vi "Append Image.vi"(1 "Cell Address":string, 4 "Image Path":path, 6 "error in (no error)":errorcluster, 7 "Column Index":i32, 8 "Caption":string, 9 "Row Index":i32, 10 "Report Ref In":T2) -> (0 "error out":errorcluster, 2 "Image Index":i32, 3 "Report Ref Out":T2)   [LabVIEW 2026, in "XCel Report Engine.lvlib"]
uses:
  XCel Report Engine.lvlib
  Controls/Report Ref.ctl
  C:/Users/m.santucci/Documents/ChatGPT/LV_REPORT_ENGINE/.net/src/XCelReportEngine/bin/Release/net48/XCelReportEngine.dll
  .net/src/XCelReportEngine/bin/Release/net48/XCelReportEngine.dll
  Controls/Image Alignment.ctl
panel:
  in  "Image Alignment":T1
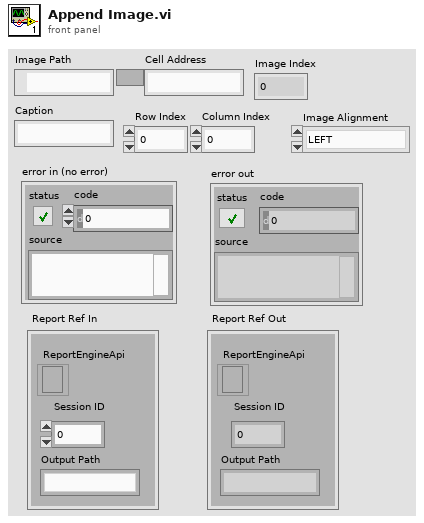
[diagram p1: front panel]
types:
  T1 = typedef "XCel Report Engine.lvlib/Image Alignment.ctl" = enum32{"LEFT", "RIGHT", "TOP", "TEXTTOP", "MIDDLE", "ABSMIDDLE", "BASELINE", "BOTTOM", "ABSBOTTOM"}
  T2 = typedef "XCel Report Engine.lvlib/Report Ref.ctl" = cluster{"Session ID":i32, "Output Path":string, "ReportEngineApi":refnum<k24>}
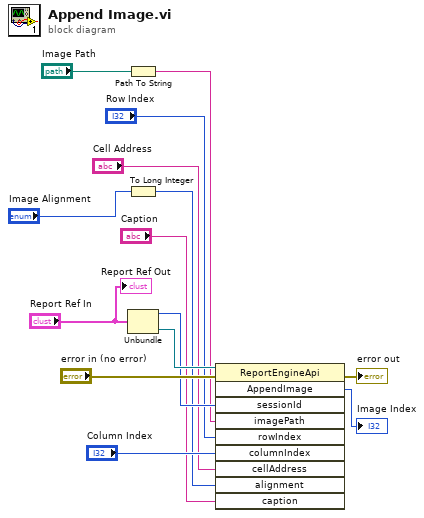
[diagram p0: block diagram]
diagram:
  n1 = Path To String(path="Image Path") -> (string=w6:string)
  n2 = To Long Integer(number="Image Alignment") -> (32bit integer=w2:i32)
  n3 = Unbundle("Report Ref In") -> ("Session ID"=w10:i32, "ReportEngineApi"=w13:refnum<k24>)  [unwired: 1 out]
  n4 = invoke class="ReportEngineApi" method="AppendImage"(reference=w13, error in="error in (no error)", "sessionId"=w10, "imagePath"=w6, "rowIndex"="Row Index", "columnIndex"="Column Index", "cellAddress"="Cell Address", "alignment"=w2, "caption"="Caption") -> (error out=→"error out":errorcluster, "AppendImage"=→"Image Index":i32)  [unwired: 1 in, 8 out]
  "Report Ref Out" <- "Report Ref In"
